vi "字符串连接显示.vi"() -> ()   [LabVIEW 2018]
panel:
  out "字符串":string
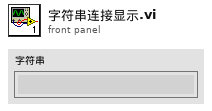
[diagram p1: front panel]
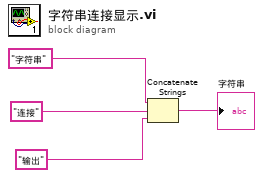
[diagram p0: block diagram]
diagram:
  n1 = Concatenate Strings("字符串", "连接", "输出") -> (→"字符串":string)
